vi "Acquire Data.vi"(0 "Number of Samples":i32, 1 "Desired Sample Rate (Hz)":dbl, 2 "Minimum Value":dbl, 3 "Maximum Value":dbl, 4 "Physical Channels":tag, 5 "error in":errorcluster) -> (14 "Data Out":dbl[][](array[numeric]) format="%0.2f", 15 "Actual Sample Rate (Hz)":dbl, 19 "error out":errorcluster)   [LabVIEW 2021]
uses:
  <vilib>/DAQmx/read.llb/DAQmx Read (Analog 2D DBL NChan NSamp).vi
  <vilib>/DAQmx/create/channels.llb/DAQmx Create Channel (AI-Voltage-Basic).vi
  <vilib>/DAQmx/configure/timing.llb/DAQmx Timing (Sample Clock).vi
  <vilib>/DAQmx/miscellaneous.llb/DAQmx Fill In Error Info.vi
  <resource>/objmgr/daqmx.rc
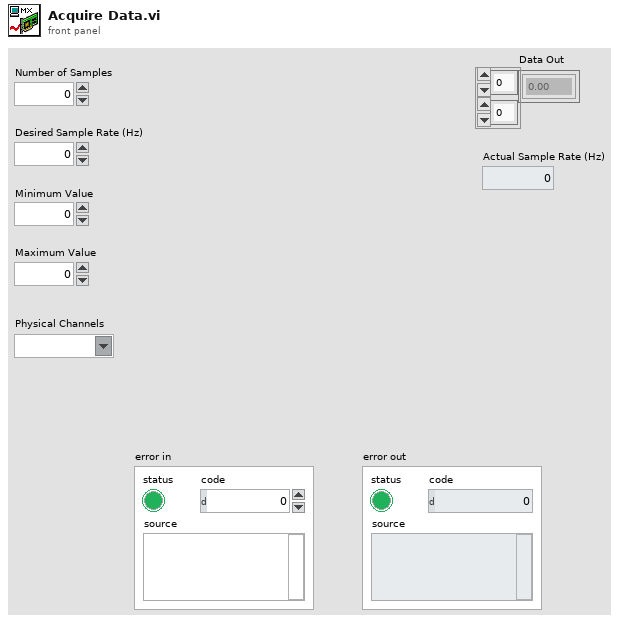
[diagram p1: front panel]
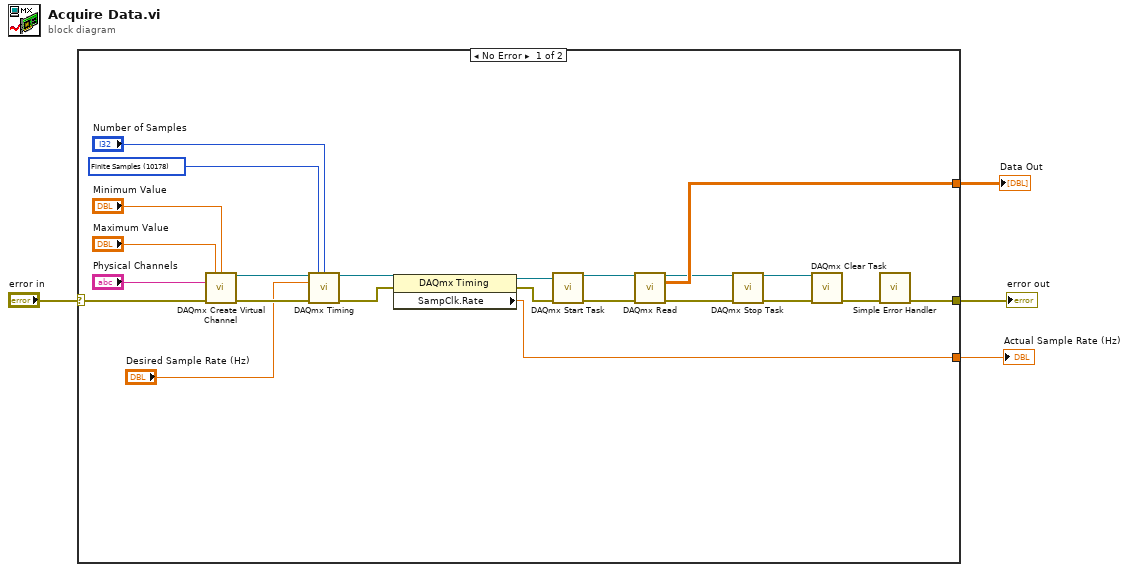
[diagram p0: block diagram]
diagram:
  n1 = case shown="No Error" "error in" {
    selector: "error in" -> [w27 w28]
    tunnel: [w17 w28] -> w3
    tunnel: [w19 _] -> w2
    tunnel: [w18 _] -> w1
    frame No Error {
      w12 = 10178 items=["Finite Samples"=10178, "Continuous Samples"=10123, "Hardware Timed Single Point"=12522] ("sample mode")
      n2 = call-poly <vilib>:"DAQmx Create Virtual Channel.vi"("maximum value"="Maximum Value", "minimum value"="Minimum Value", "physical channels"="Physical Channels", "error in"=w27) -> ("task out"=w10:refnum<k21>, "error out"=w26:errorcluster)  [unwired: 10 in]
      n3 = call-poly <vilib>:"DAQmx Timing.vi"("task/channels in"=w10, "sample mode"=w12, "samples per channel"="Number of Samples", "rate"="Desired Sample Rate (Hz)", "error in"=w26) -> ("task out"=w9:refnum<k21>, "error out"=w25:errorcluster)  [unwired: 9 in]
      n4 = property class="DAQmx Timing"(reference=w9, error in=w25) -> (reference out=w8:refnum<k21>, error out=w24:errorcluster, "SampClk.Rate"=w18:dbl)
      n5 = call <vilib>:"DAQmx Start Task.vi"("task/channels in"=w8, "error in"=w24) -> ("task out"=w7:refnum<k21>, "error out"=w23:errorcluster)  [unwired: 12 in]
      n6 = call-poly <vilib>:"DAQmx Read.vi"("task/channels in"=w7, "error in"=w23) -> ("task out"=w6:refnum<k21>, "data"=w19:dbl[][], "error out"=w22:errorcluster)  [unwired: 11 in]
      n7 = call <vilib>:"DAQmx Stop Task.vi"("task/channels in"=w6, "error in"=w22) -> ("task out"=w5:refnum<k21>, "error out"=w21:errorcluster)  [unwired: 12 in]
      n8 = call <vilib>:"DAQmx Clear Task.vi"("task in"=w5, "error in"=w21) -> ("error out"=w20:errorcluster)  [unwired: 13 in]
      n9 = call <vilib>:"Simple Error Handler.vi"("error in (no error)"=w20) -> ("error out"=w17:errorcluster)  [unwired: 4 in, 4 out]
    }
    frame Error {
    }
  }
  "error out" <- w3
  "Actual Sample Rate (Hz)" <- w1
  "Data Out" <- w2
